vi "GUI_Plasma1_pressure_cal1.vi"() -> ()   [LabVIEW 2013]
uses:
  Shared/GUI_Template/GUI_master/tcp_new_data_event.ctl
  Shared/GUI_Template/GUI_master/tcp new data cluster.ctl
panel:
  out "pressure chart 2":dbl(graph) caption="PR4000 pressure"
  out "flow::11":dbl=25.5 caption="PR4000 Flow" min=0.0 max=0.0 format="%_4f"
  in  "valve::11":bool caption="Valve"
  in  "pressure::11":dbl=25.5 caption="PR4000 Pressure" min=0.0 max=200.0 format="%_4f"
  in  "pressure::9":dbl=25.5 caption="Baratron Pressure" min=-100.0 max=500.0 format="%_4f"
  out "pressure chart":dbl(graph) caption="Baratron pressure"
  in  "GUIdevice 11":string="BELLA_LowPressureControl"
  in  "GUIdevice 9":string="BELLA_PDR2000"
  out "error IO 2":errorcluster
  in  "insert tag":bool=TRUE
  out "tcp data event":T1
  in  "stop":bool
  in  "UDP error message":string
  # "Plasma 1 Pressure calibration VI"
  # "Pressures"
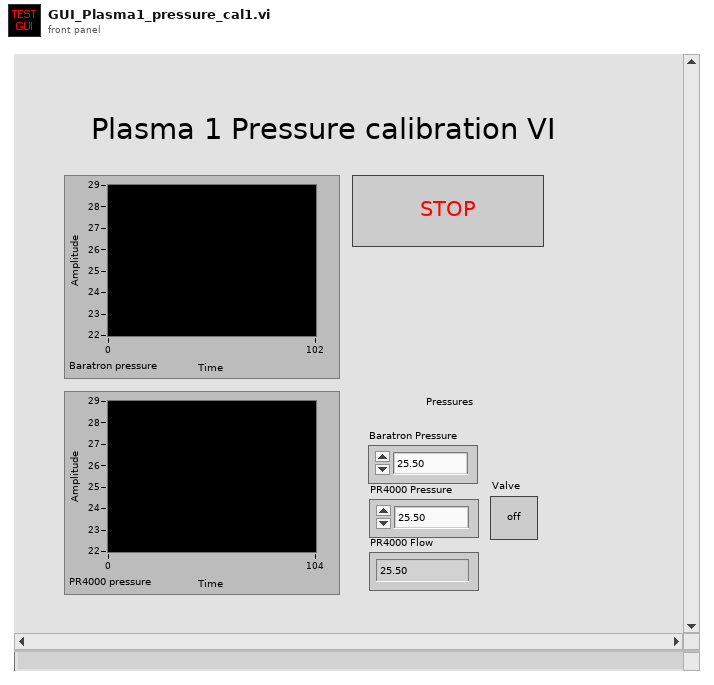
[diagram p1: front panel]
types:
  T1 = typedef "tcp_new_data_event.ctl" = refnum<user-event>
  T2 = typedef "tcp new data cluster.ctl" = cluster{"EventEnum":enum16{"new data", "connection status update"}, "Device name":string}
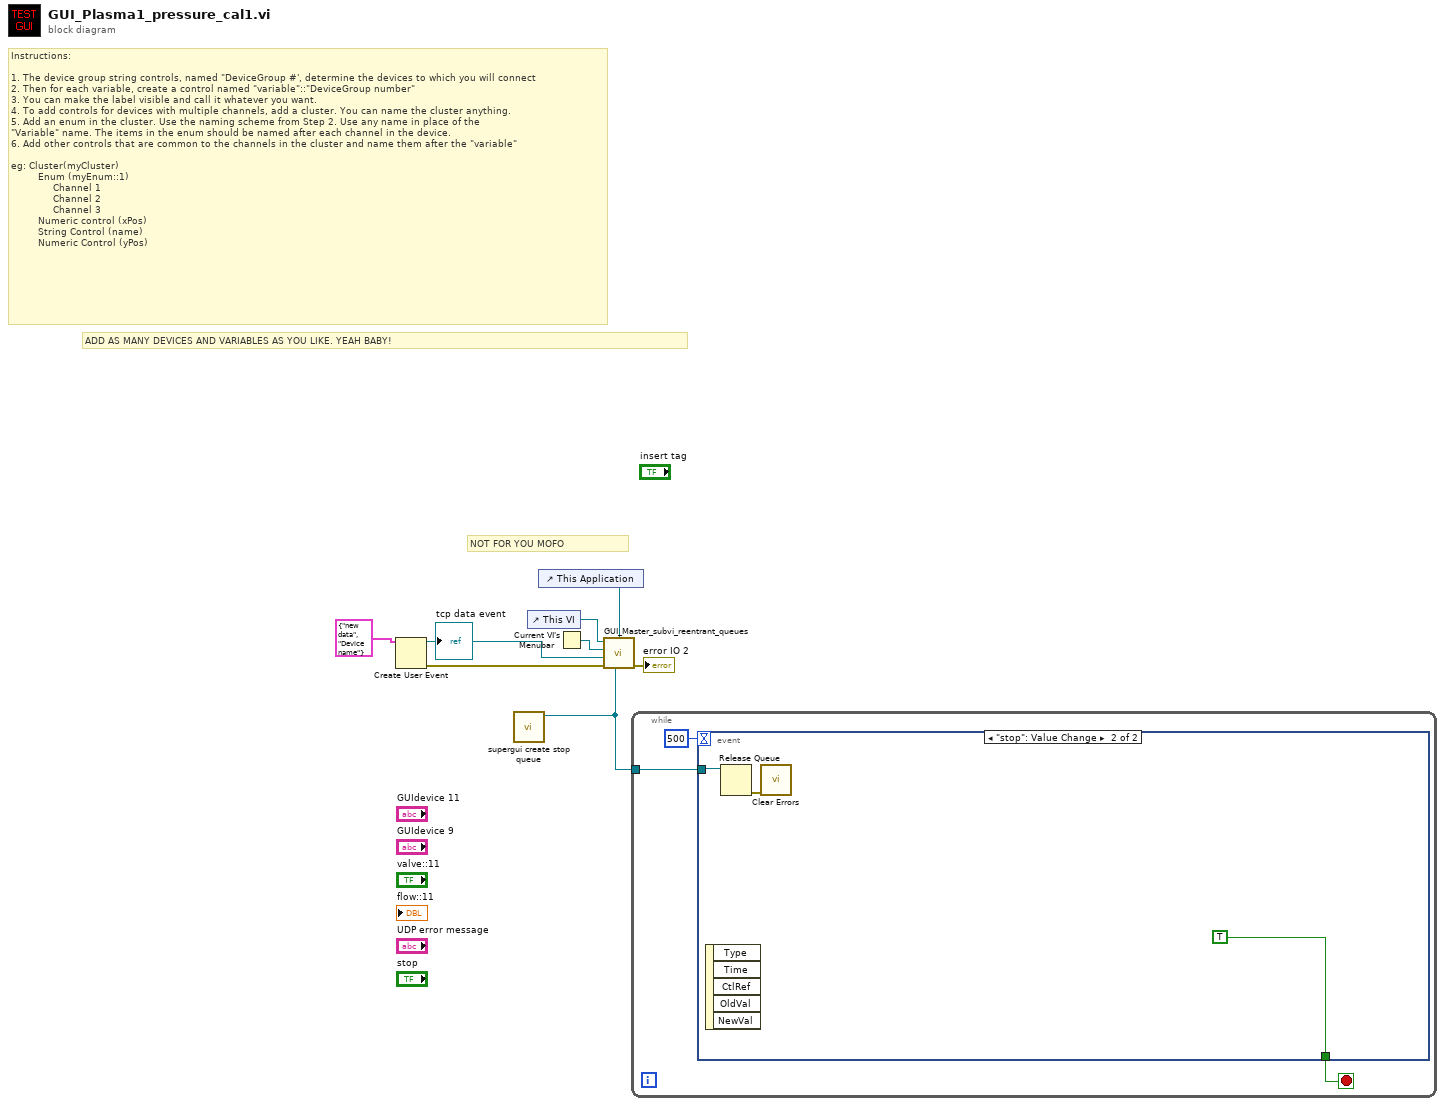
[diagram p0: block diagram]
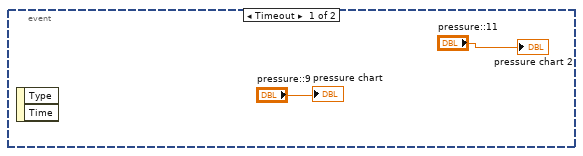
[diagram p2: hidden frame]
diagram:
  # "Instructions:\n\n1. The device group string controls, named \"DeviceGroup #', determine the devices to which you will connect\n2. Then for each variable, create a control named \"variable\"::\"DeviceGroup number\"\n3. You can make the label visible and call it whatever you want.\n4. To add controls for devices with multiple channels, add a cluster. You can name the cluster anything.\n5. Add an enum in the cluster. Use the naming scheme from Step 2. Use any name in place of the \n\"Variable\" name. The items in the enum should be named after each channel in the device. \n6. Add other controls that are common to the channels in the cluster and name them after the \"variable\"\n\neg: Cluster(myCluster)\n         Enum (myEnum::1)\n              Channel 1 \n              Channel 2\n              Channel 3\n         Numeric control (xPos)\n         String Control (name)\n         Numeric Control (yPos)"
  # "ADD AS MANY DEVICES AND VARIABLES AS YOU LIKE. YEAH BABY!"
  # "NOT FOR YOU MOFO"
  n1 = Create User Event(user event datatype=T2 {"EventEnum"=enum."new data", "Device name"="Device name"} ("New Event")) -> (user event=w3:refnum<user-event>, error out=w8:errorcluster)  [unwired: 1 in]
  "tcp data event" <- w3
  n2 = call "supergui create stop queue.vi"() -> ("STOP Queue out"=w1:refnum<queue>)  [unwired: 11 in]
  n3 = control-ref of="This VI"() -> (w5:refnum<vi>)
  n4 = control-ref of="This Application"() -> (w2:refnum<vi>)
  n5 = Current VI's Menubar() -> (w6:refnum<k9>)
  n6 = call "GUI_Master_subvi_reentrant_queues.vi"("STOP Queue in"=w1, "This Application"=w2, "error in (no error)"=w8, "tcp data event"=w3, "Caller menu reference"=w6, "Caller VI ref"=w5) -> ("error out"=→"error IO 2":errorcluster)  [unwired: 5 in]
  n7 = while {
    tunnel: w1 -> [w9]
    stop <- w10 stop-if-true
    n8 = event shown="[1] \"stop\": Value Change" {
      selector: _ -> [_ _]
      dyn-events: _ -> [_ _]
      timeout: 500 -> [_ _]
      tunnel: [_ TRUE] -> w10
      tunnel: w9 -> [_ w15]
      event Timeout {
        n9 = event-data() -> ()  [unwired: 1 in, 2 out]
        "pressure chart" <- "pressure::9"
        "pressure chart 2" <- "pressure::11"
      }
      event "stop": Value Change {
        n10 = event-data() -> ()  [unwired: 1 in, 5 out]
        n11 = Release Queue(queue=w15) -> (error out=w14:errorcluster)  [unwired: 2 in, 2 out]
        n12 = call <vilib>:"Clear Errors.vi"("error in (no error)"=w14) -> ()  [unwired: 6 in, 1 out]
      }
    }
  }
